vi "WPI_CounterGet.vi"(8 "error in (no error)":errorcluster, 11 "CounterDevRef in":T1) -> (0 "error out":errorcluster, 1 "Direction":bool, 2 "Value":i32, 3 "CounterDevRef out":T1, 4 "Period (sec)":dbl, 6 "Stopped":bool)   [LabVIEW 2017]
doc: "Returns information, such as number of counts and the period, from the counter you specify.\n\nThis software is licensed. Open the labview\\readme\\WPI Robotics Library Open Source License.txt file for more information."
uses:
  <vilib>/Rock Robotics/WPI/Counter/WPI_CounterDevRef.ctl
  <vilib>/Rock Robotics/SystemInterfaces/Counter/FPGA_CounterCtrSystemIndex.ctl
  <vilib>/Rock Robotics/SystemInterfaces/Counter/FPGA_CounterERRInvalidResource.vi
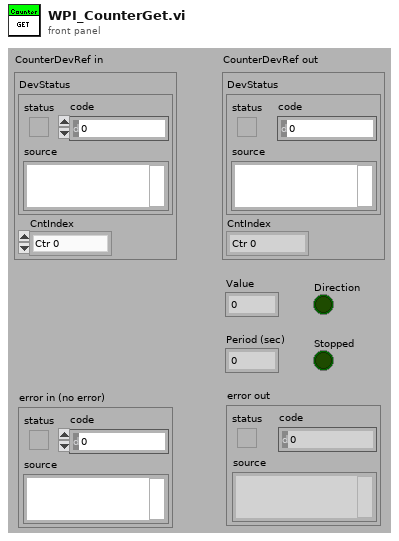
[diagram p1: front panel]
types:
  T1 = typedef "WPI_CounterDevRef.ctl" = cluster{"DevStatus":errorcluster, "CntIndex":T2}
  T2 = typedef "FPGA_CounterCtrSystemIndex.ctl" = enum8{"Ctr 0", "Ctr 1", "Ctr 2", "Ctr 3", "Ctr 4", "Ctr 5", "Ctr 6", "Ctr 7", "Invalid"}
  T3 = typedef "FPGA_CounterCtrDevRef.ctl" = cluster{"DevStatus":errorcluster, "CntIndex":T2}
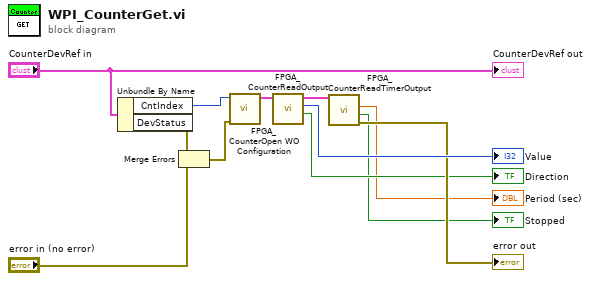
[diagram p0: block diagram]
diagram:
  n1 = Unbundle By Name("CounterDevRef in") -> ("CntIndex"=w6:T2, "DevStatus"=w3:errorcluster)
  n2 = Merge Errors(w3, "error in (no error)") -> (w2:errorcluster)
  n3 = call <vilib>:"FPGA_CounterOpen WO Configuration.vi"("error in"=w2, "CntIndex"=w6) -> ("Ctr Ref"=w5:T3)  [unwired: 1 in, 8 out]
  n4 = call <vilib>:"FPGA_CounterReadOutput.vi"("Ctr Ref in"=w5) -> ("Direction"=→"Direction":bool, "Value"=→"Value":i32, "Ctr Ref out"=w4:T3)  [unwired: 1 in, 7 out]
  n5 = call <vilib>:"FPGA_CounterReadTimerOutput.vi"("Ctr Ref in"=w4) -> ("error out"=→"error out":errorcluster, "Stalled"=→"Stopped":bool, "Period (s)"=→"Period (sec)":dbl)  [unwired: 1 in, 7 out]
  "CounterDevRef out" <- "CounterDevRef in"
